vi "Laserpaneltcp.vi"() -> ()   [LabVIEW 2014]
uses:
  wlmData.dll
panel:
  out "Boolean 2":bool
  out "Boolean":bool
  in  "Warning 3":bool
  in  "Warning 2":bool
  in  "Warning 1":bool
  in  "Warning 0":bool
  out "Set Volt Array 0":dbl[](array[numeric])
  out "935":string
  out "729":string
  out "399":string
  out "370":string
  out "Act Wavelength number (nm)":dbl=70.0 format="%.6f"
  out "Set wave Array":dbl[](array[numeric])
  out "Lock Array":bool[](array[boolean])
  in  "stop":bool
  in  "Tab Control":enum32{"Laser Controller", "Wavelenth Meter"}(tab)
  out "Act Temperature":dbl=70.0 format="%.3f"
  out "Max Current (mA)":dbl=70.0 format="%.3f"
  out "Act Current (mA)":dbl=70.0 format="%.1f"
  in  "Set Wavelength (nm)":dbl=935.1882 format="%.6f"
  in  "Lock":bool
  in  "Laser":i16(ring) items=["370", "399", "729", "935"]
  out "Act Voltage (V)":dbl=70.0 format="%.3f"
  in  "Set Temperature":dbl=70.0 format="%.3f"
  in  "Set Current  (mA)":dbl=70.0 format="%.3f"
  in  "Set Voltage (V)":dbl=70.0 format="%.3f"
  out "Warning":bool
  in  "PID gains":T1={"proportional gain (Kc)"=1000.0, "integral time (Ti, min)"=0.0, "derivative time (Td, min)"=0.0} {"derivative time (Td, min)" format="%.3f"; "integral time (Ti, min)" format="%.3f"; "proportional gain (Kc)" format="%.3f"}
  out "Act Wavelength (nm)":string
  in  "PID Warning":bool
  in  "stop 3":bool
  in  "Use":bool=TRUE
  in  "Use":bool=TRUE
  in  "Use":bool=TRUE
  in  "Use":bool=TRUE
  in  "Expo.4[ms]":i32[](array[numeric])
  in  "Expo.3[ms]":i32[](array[numeric])
  in  "Expo.2[ms]":i32[](array[numeric])
  out "935 2":string
  out "729  2":string
  out "399 2":string
  out "370 2":string
  in  "Show":bool=TRUE
  in  "Show":bool=TRUE
  in  "Show":bool=TRUE
  in  "Show":bool=TRUE
  in  "Automatic":bool
  in  "Automatic":bool
  in  "Automatic":bool
  in  "Automatic":bool
  out "Pattern2":i16[][](graph)
  out "Pattern":i16[][](graph)
  in  "Expo.1[ms]":i32[](array[numeric])
  in  "stop 2":bool
  in  "Show WLM APP":bool=TRUE
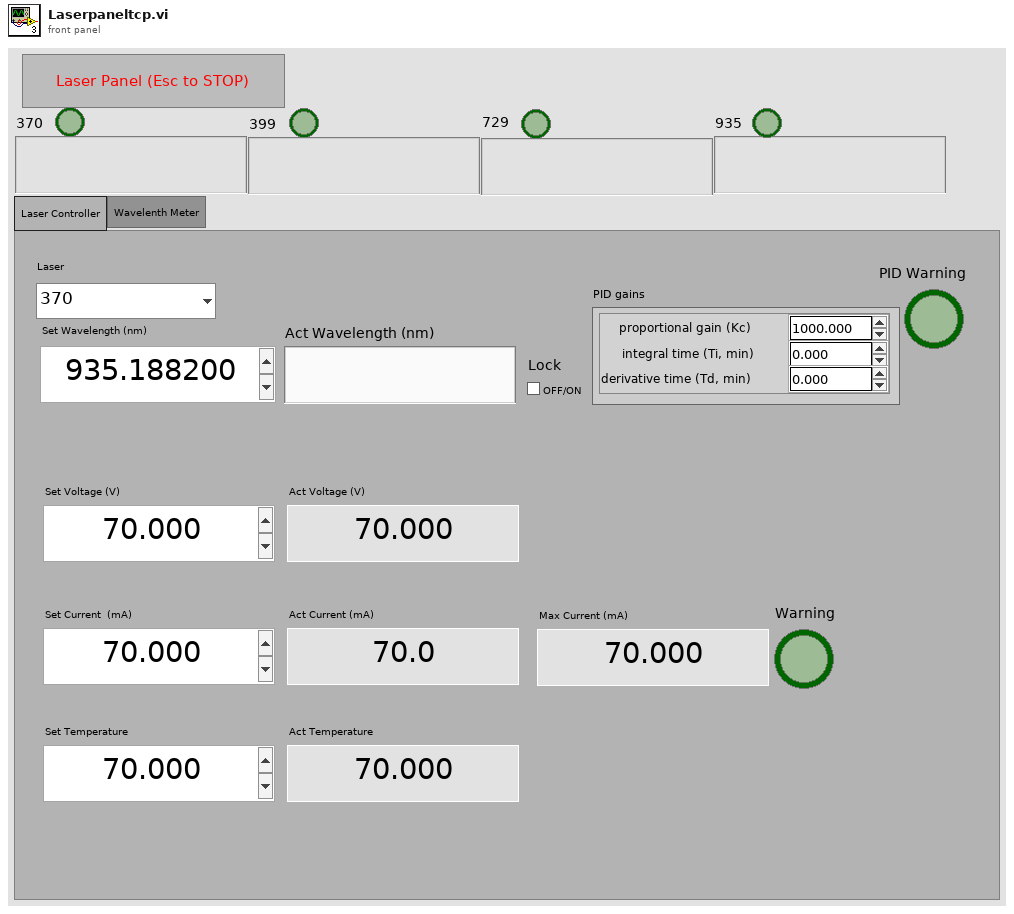
[diagram p1: front panel]
types:
  T1 = cluster{"proportional gain (Kc)":dbl, "integral time (Ti, min)":dbl, "derivative time (Td, min)":dbl}
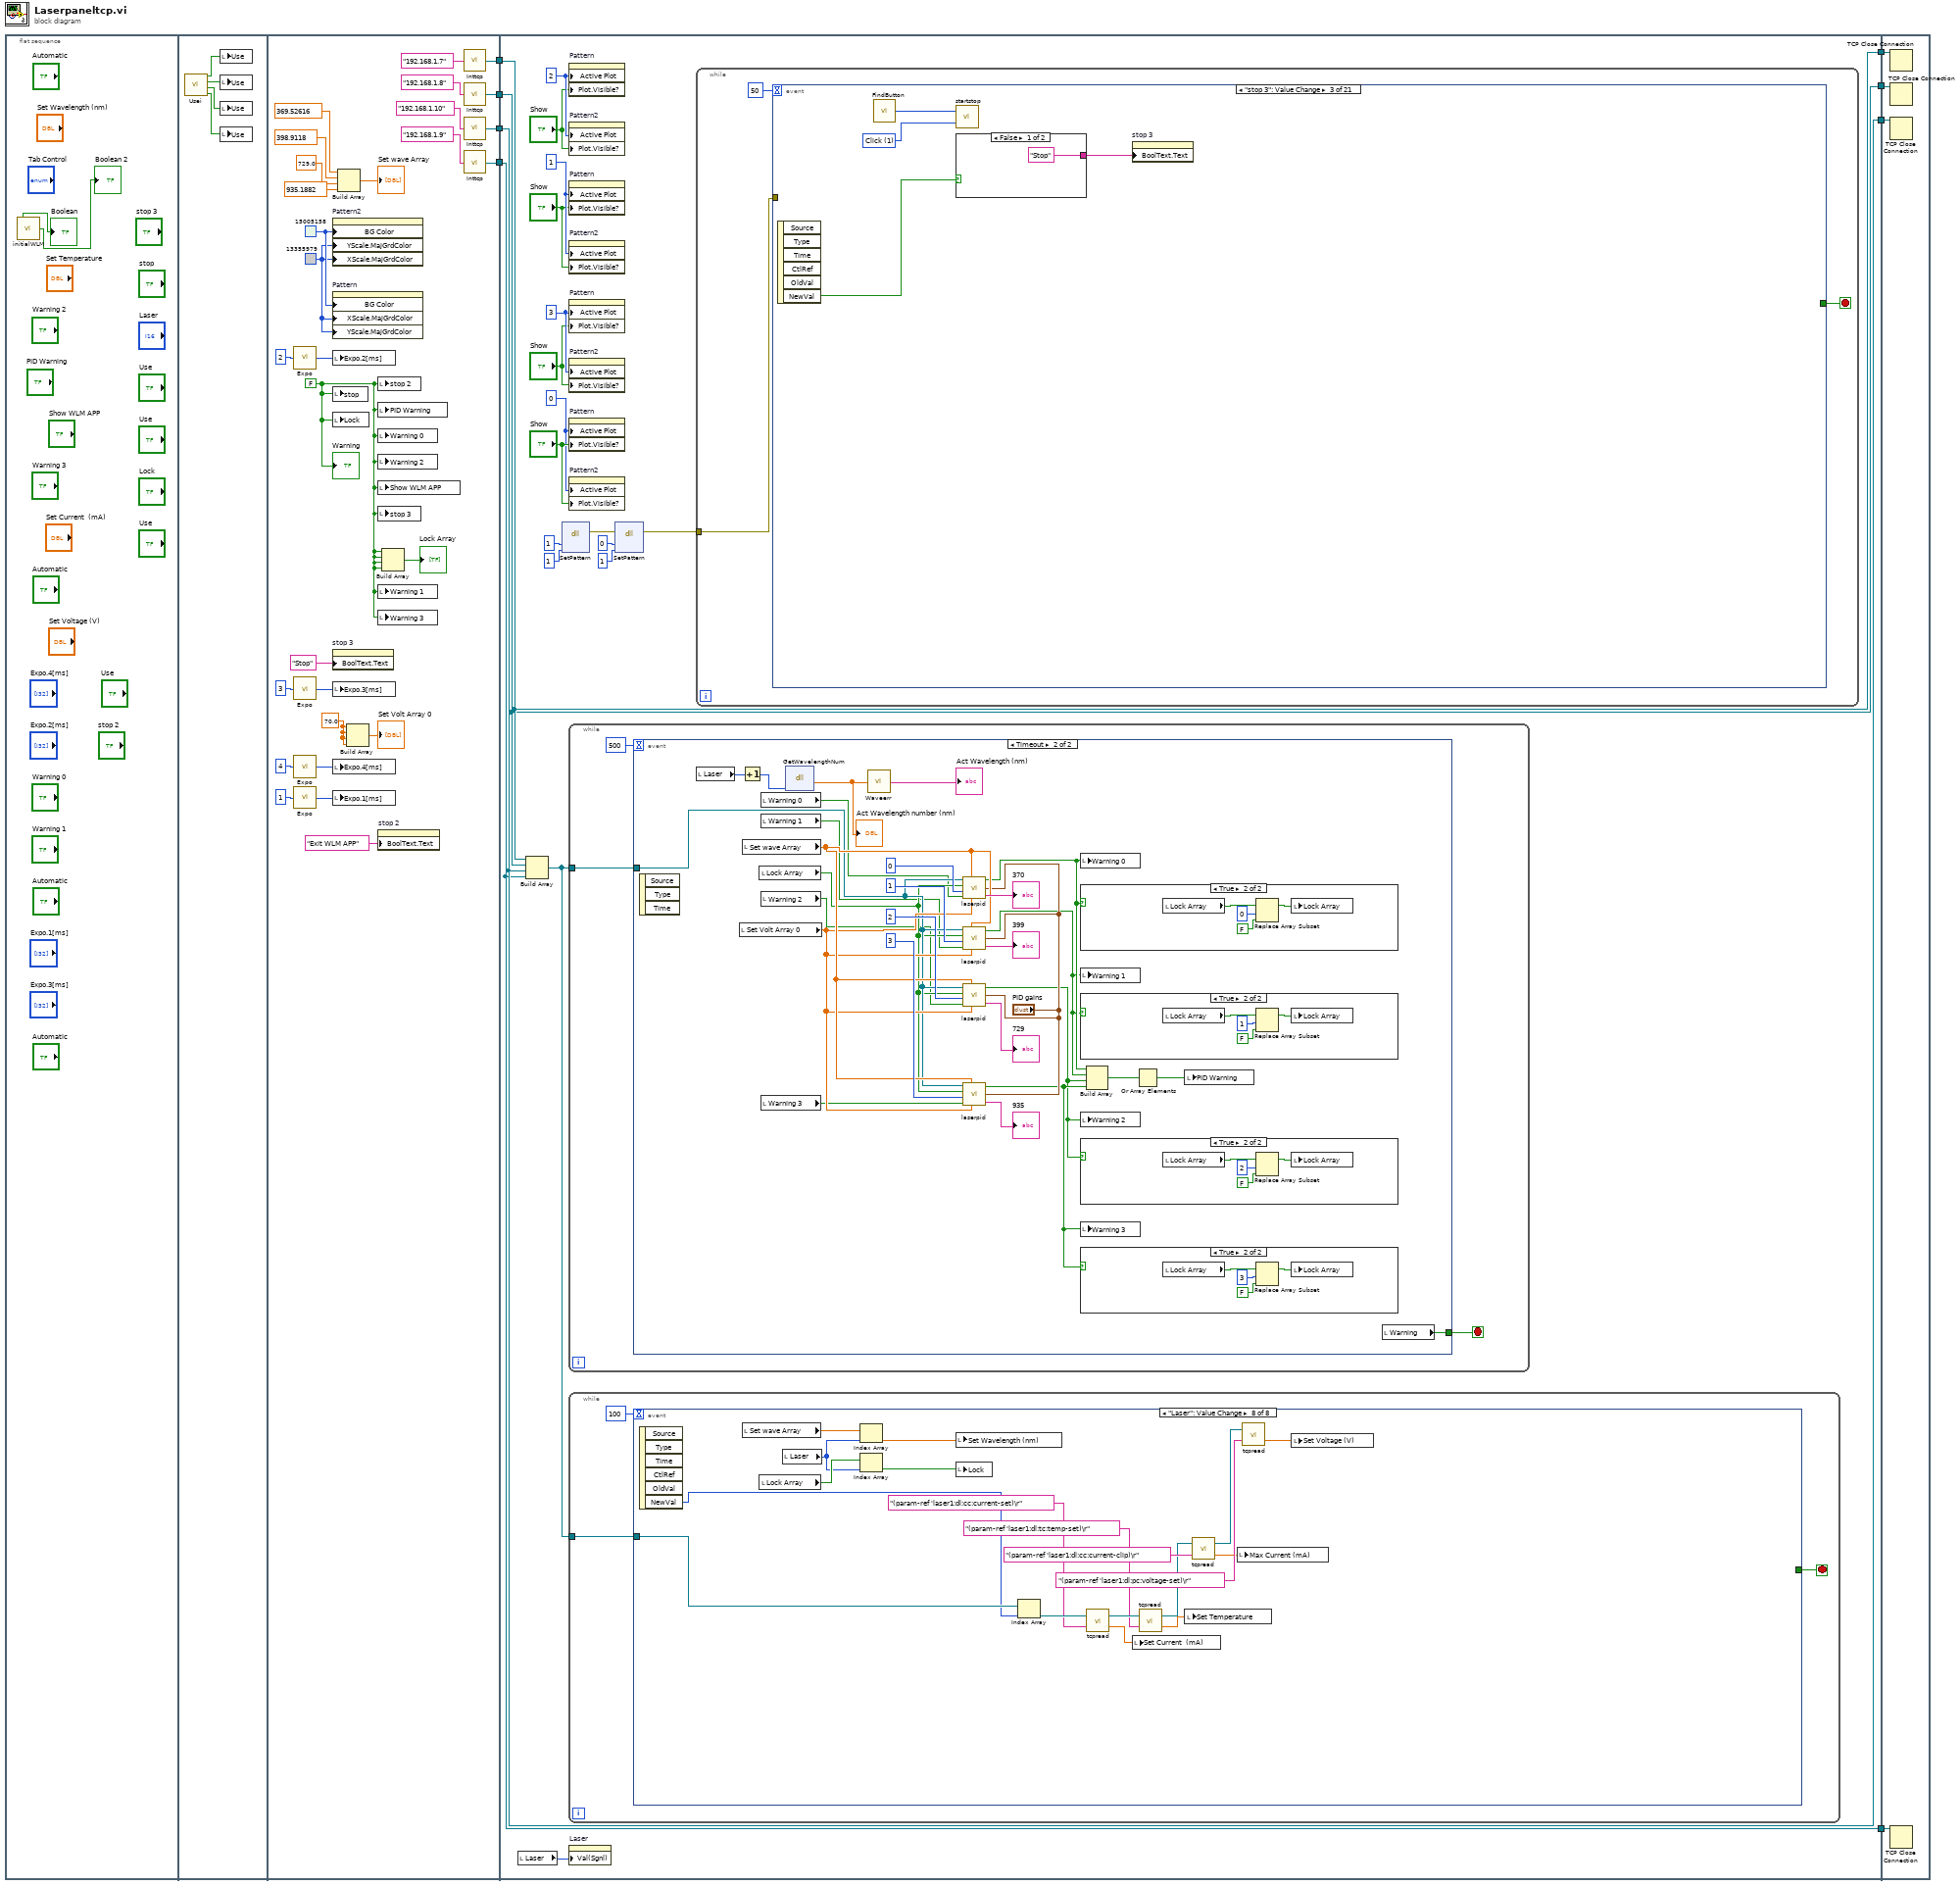
[diagram p0: block diagram]
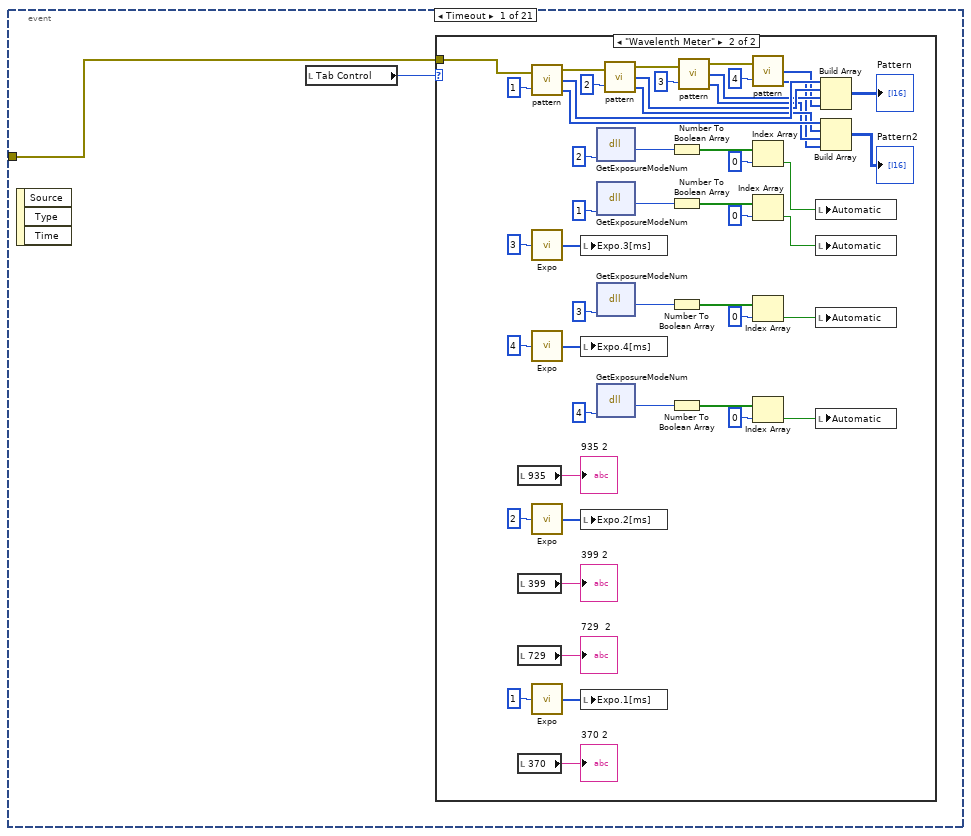
[diagram p2: hidden frame]
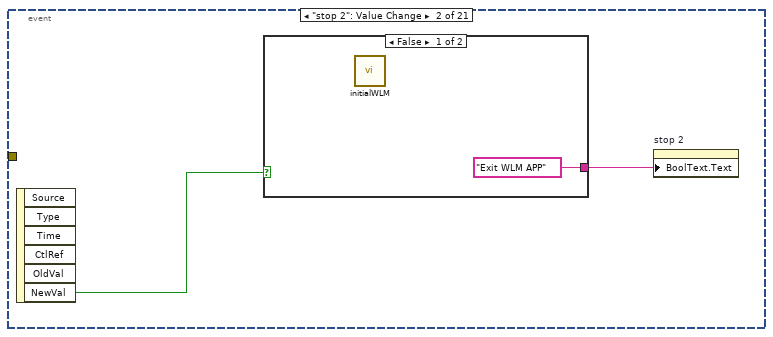
[diagram p4: hidden frame]
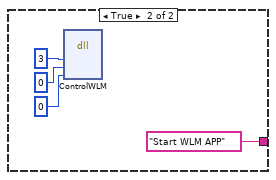
[diagram p5: hidden frame]
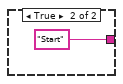
[diagram p6: hidden frame]
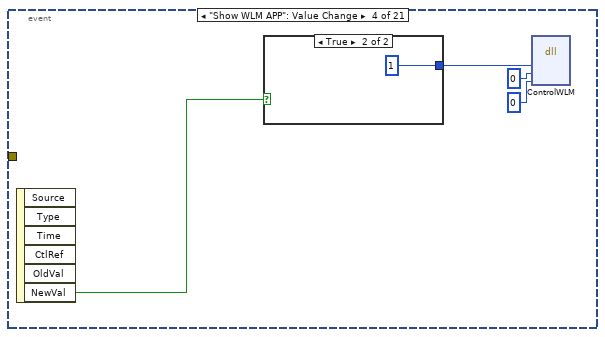
[diagram p7: hidden frame]
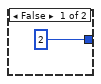
[diagram p8: hidden frame]
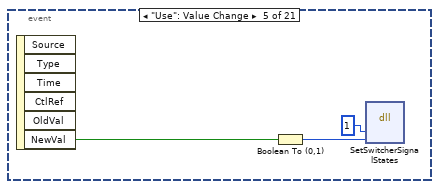
[diagram p9: hidden frame]
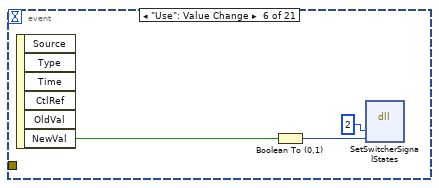
[diagram p10: hidden frame]
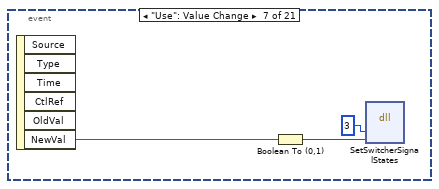
[diagram p11: hidden frame]
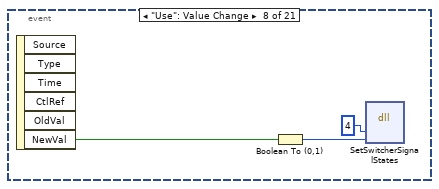
[diagram p12: hidden frame]
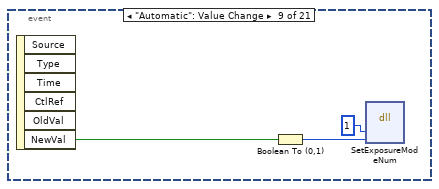
[diagram p13: hidden frame]
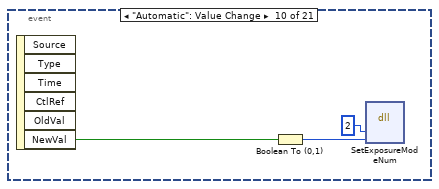
[diagram p14: hidden frame]
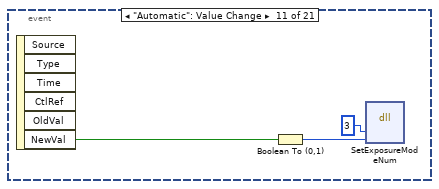
[diagram p15: hidden frame]
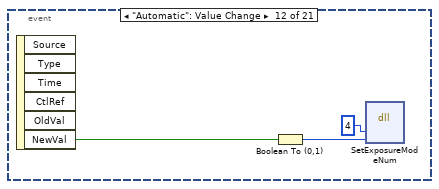
[diagram p16: hidden frame]
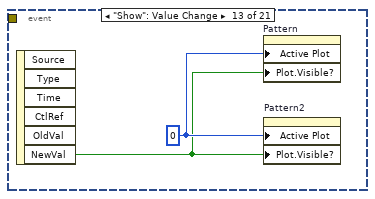
[diagram p17: hidden frame]
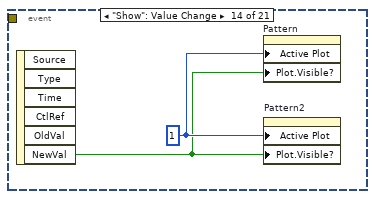
[diagram p18: hidden frame]
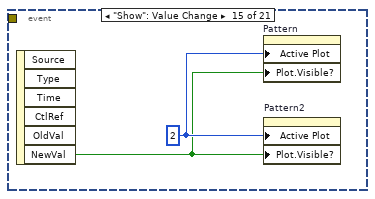
[diagram p19: hidden frame]
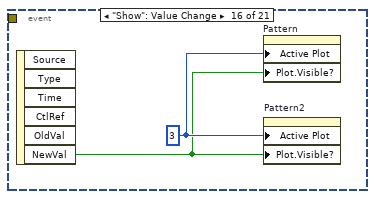
[diagram p20: hidden frame]
diagram:
  n1 = flat-sequence {
    tunnel: [w41] -> w8
    tunnel: [w40] -> w7
    tunnel: [w39] -> w6
    tunnel: [w38] -> w5
    tunnel: w8 -> [w62]
    tunnel: w7 -> [w61]
    tunnel: w6 -> [w60]
    tunnel: w5 -> [w59]
    tunnel: [w62] -> w4
    tunnel: [w61] -> w3
    tunnel: [w60] -> w2
    tunnel: [w59] -> w1
    tunnel: w4 -> [w360]
    tunnel: w3 -> [w359]
    tunnel: w2 -> [w358]
    tunnel: w1 -> [w357]
    frame #0 {
      n2 = call "initialWLM.vi"() -> ("Boolean 2"=→"Boolean 2":bool, "Boolean"=→"Boolean":bool)
    }
    frame #1 {
      n3 = call "Usei.vi"() -> ("Boolean 4"=w14:bool, "Boolean 3"=w13:bool, "Boolean 2"=w12:bool, "Boolean"=w11:bool)
      n4 = local write "Use"(w11) -> ()
      n5 = local write "Use"(w12) -> ()
      n6 = local write "Use"(w13) -> ()
      n7 = local write "Use"(w14) -> ()
    }
    frame #2 {
      w26 = u32 13355979 ("Color Box")
      w27 = u32 15005158
      w30 = 70.0
      w17 = FALSE
      n8 = call "Expo.vi"("Numeric"=2) -> ("Array"=w22:i32[])
      n9 = call "Expo.vi"("Numeric"=3) -> ("Array"=w20:i32[])
      n10 = call "Expo.vi"("Numeric"=4) -> ("Array"=w18:i32[])
      n11 = call "Expo.vi"("Numeric"=1) -> ("Array"=w24:i32[])
      n12 = property on="Pattern2" class="WFGraph (strict)"("BG Color"=w27, "YScale.MajGrdColor"=w26, "XScale.MajGrdColor"=w26) -> ()  [unwired: 2 in, 2 out]
      n13 = property on="Pattern" class="WFGraph (strict)"("BG Color"=w27, "XScale.MajGrdColor"=w26, "YScale.MajGrdColor"=w26) -> ()  [unwired: 2 in, 2 out]
      n14 = local write "Expo.2[ms]"(w22) -> ()
      n15 = local write "stop"(w17) -> ()
      n16 = local write "Lock"(w17) -> ()
      n17 = property on="stop 3" class="Bool (strict)"("BoolText.Text"="Stop") -> ()  [unwired: 2 in, 2 out]
      n18 = local write "Expo.3[ms]"(w20) -> ()
      n19 = local write "Expo.4[ms]"(w18) -> ()
      n20 = local write "Expo.1[ms]"(w24) -> ()
      n21 = Build Array(369.52616, 398.9118, 729.0, 935.1882) -> (→"Set wave Array":dbl[])
      n22 = Build Array(w30, w30, w30, w30) -> (→"Set Volt Array 0":dbl[])
      n23 = local write "stop 2"(w17) -> ()
      n24 = local write "PID Warning"(w17) -> ()
      n25 = local write "Warning 0"(w17) -> ()
      n26 = local write "Warning 2"(w17) -> ()
      n27 = local write "Show WLM APP"(w17) -> ()
      n28 = local write "stop 3"(w17) -> ()
      n29 = local write "Warning 1"(w17) -> ()
      n30 = local write "Warning 3"(w17) -> ()
      n31 = property on="stop 2" class="Bool (strict)"("BoolText.Text"="Exit WLM APP") -> ()  [unwired: 2 in, 2 out]
      n32 = Build Array(w17, w17, w17, w17) -> (→"Lock Array":bool[])
      n33 = call "Inttcp.vi"("String"="192.168.1.7" ("address")) -> ("TCP Network Connection Refnum"=w41:refnum<k5>)
      n34 = call "Inttcp.vi"("String"="192.168.1.8" ("address")) -> ("TCP Network Connection Refnum"=w40:refnum<k5>)
      n35 = call "Inttcp.vi"("String"="192.168.1.10" ("address")) -> ("TCP Network Connection Refnum"=w39:refnum<k5>)
      n36 = call "Inttcp.vi"("String"="192.168.1.9" ("address")) -> ("TCP Network Connection Refnum"=w38:refnum<k5>)
      "Warning" <- w17
    }
    frame #3 {
      w55 = 3
      w57 = 2
      w51 = 1
      w52 = 0
      n37 = local read "Laser"() -> (w63:i16)
      n38 = Build Array(w62, w61, w60, w59) -> (w58:refnum<k5>[])
      n39 = dll-call lib="wlmData.dll" fn="SetPattern"("Index"=1, "enable"=1) -> (error out=w45:errorcluster)  [unwired: 6 in, 1 out]
      n40 = property on="Pattern" class="WFGraph (strict)"("Active Plot"=w57, "Plot.Visible?"="Show") -> ()  [unwired: 2 in, 2 out]
      n41 = property on="Pattern2" class="WFGraph (strict)"("Active Plot"=w57, "Plot.Visible?"="Show") -> ()  [unwired: 2 in, 2 out]
      n42 = property on="Pattern" class="WFGraph (strict)"("Active Plot"=w51, "Plot.Visible?"="Show") -> ()  [unwired: 2 in, 2 out]
      n43 = property on="Pattern2" class="WFGraph (strict)"("Active Plot"=w51, "Plot.Visible?"="Show") -> ()  [unwired: 2 in, 2 out]
      n44 = property on="Pattern" class="WFGraph (strict)"("Active Plot"=w55, "Plot.Visible?"="Show") -> ()  [unwired: 2 in, 2 out]
      n45 = property on="Pattern2" class="WFGraph (strict)"("Active Plot"=w55, "Plot.Visible?"="Show") -> ()  [unwired: 2 in, 2 out]
      n46 = property on="Pattern" class="WFGraph (strict)"("Active Plot"=w52, "Plot.Visible?"="Show") -> ()  [unwired: 2 in, 2 out]
      n47 = property on="Pattern2" class="WFGraph (strict)"("Active Plot"=w52, "Plot.Visible?"="Show") -> ()  [unwired: 2 in, 2 out]
      n48 = while {
        tunnel: w58 -> [w205]
        stop <- w206 stop-if-true
        n49 = event shown="[1] Timeout" {
          selector: _ -> [_ _]
          dyn-events: _ -> [_ _]
          timeout: 500 -> [_ _]
          tunnel: [w208 w219] -> w206
          tunnel: w205 -> [_ w222]
          event "stop": Value Change {
            n50 = event-data() -> ("NewVal"=w208:bool)  [unwired: 1 in, 5 out]
          }
          event Timeout {
            n51 = event-data() -> ()  [unwired: 1 in, 3 out]
            n52 = local read "Laser"() -> (w233:i16)
            n53 = local read "Set Volt Array 0"() -> (w223:dbl[])
            n54 = Increment(x=w233) -> (x+1=w234:i16)
            n55 = local read "Set wave Array"() -> (w224:dbl[])
            n56 = local read "Lock Array"() -> (w221:bool[])
            n57 = local read "Warning 0"() -> (w218:bool)
            n58 = local read "Warning 1"() -> (w217:bool)
            n59 = local read "Warning 2"() -> (w216:bool)
            n60 = local read "Warning 3"() -> (w215:bool)
            n61 = dll-call lib="wlmData.dll" fn="GetWavelengthNum"("channel"=w234) -> ("res"=w235:dbl)  [unwired: 4 in, 2 out]
            "Act Wavelength number (nm)" <- w235
            n62 = call "Waveerr.vi"("Numeric"=w235) -> ("String"=→"Act Wavelength (nm)":string)
            n63 = call "laserpid.vi"("TCP Array"=w222, "Set wave Array"=w224, "Lock Array"=w221, "Numeric"=0, "Set volt Array 0"=w223, "waring in"=w218, "PID gains"="PID gains") -> ("warning out"=w214:bool, "wavelenth"=→"370":string)
            n64 = call "laserpid.vi"("TCP Array"=w222, "Set wave Array"=w224, "Lock Array"=w221, "Numeric"=1, "Set volt Array 0"=w223, "waring in"=w217, "PID gains"="PID gains") -> ("warning out"=w213:bool, "wavelenth"=→"399":string)
            n65 = call "laserpid.vi"("TCP Array"=w222, "Set wave Array"=w224, "Lock Array"=w221, "Numeric"=2, "Set volt Array 0"=w223, "waring in"=w216, "PID gains"="PID gains") -> ("warning out"=w211:bool, "wavelenth"=→"729":string)
            n66 = call "laserpid.vi"("TCP Array"=w222, "Set wave Array"=w224, "Lock Array"=w221, "Numeric"=3, "Set volt Array 0"=w223, "waring in"=w215, "PID gains"="PID gains") -> ("warning out"=w212:bool, "wavelenth"=→"935":string)
            n67 = local write "Warning 0"(w214) -> ()
            n68 = case shown="True" w214 {
              frame False {
              }
              frame True {
                n69 = local read "Lock Array"() -> (w243:bool[])
                n70 = Replace Array Subset(array=w243, new element=FALSE, index=0) -> (w242:bool[])
                n71 = local write "Lock Array"(w242) -> ()
              }
            }
            n72 = local write "Warning 1"(w213) -> ()
            n73 = case shown="True" w213 {
              frame False {
              }
              frame True {
                n74 = local read "Lock Array"() -> (w251:bool[])
                n75 = Replace Array Subset(array=w251, new element=FALSE, index=1) -> (w250:bool[])
                n76 = local write "Lock Array"(w250) -> ()
              }
            }
            n77 = local write "Warning 2"(w211) -> ()
            n78 = case shown="True" w211 {
              frame False {
              }
              frame True {
                n79 = local read "Lock Array"() -> (w248:bool[])
                n80 = Replace Array Subset(array=w248, new element=FALSE, index=2) -> (w247:bool[])
                n81 = local write "Lock Array"(w247) -> ()
              }
            }
            n82 = local write "Warning 3"(w212) -> ()
            n83 = case shown="True" w212 {
              frame False {
              }
              frame True {
                n84 = local read "Lock Array"() -> (w240:bool[])
                n85 = Replace Array Subset(array=w240, new element=FALSE, index=3) -> (w239:bool[])
                n86 = local write "Lock Array"(w239) -> ()
              }
            }
            n87 = Build Array(w214, w213, w211, w212) -> (w210:bool[])
            n88 = Or Array Elements(Boolean array=w210) -> (logical OR=w209:bool)
            n89 = local write "PID Warning"(w209) -> ()
            n90 = local read "Warning"() -> (w219:bool)
          }
        }
      }
      n91 = while {
        tunnel: w58 -> [w253]
        stop <- w255 stop-if-true
        n92 = event shown="[7] \"Laser\": Value Change" {
          selector: _ -> [_ _ _ _ _ _ _ _]
          dyn-events: _ -> [_ _ _ _ _ _ _ _]
          timeout: 100 -> [_ _ _ _ _ _ _ _]
          tunnel: [w256 _ w270 _ _ _ _ _] -> w255
          tunnel: w253 -> [_ w259 w279 w284 _ w322 w331 w356]
          event "stop": Value Change {
            n93 = event-data() -> ("NewVal"=w256:bool)  [unwired: 1 in, 5 out]
          }
          event "Set Voltage (V)": Value Change {
            n94 = event-data() -> ("NewVal"=w261:dbl)  [unwired: 1 in, 5 out]
            n95 = Number To Fractional String(number=w261) -> (F-format string=w264:string)  [unwired: 3 in]
            n96 = local read "Laser"() -> (w260:i16)
            n97 = Concatenate Strings("(param-set! 'laser1:dl:pc:voltage-set " ("string"), w264, ")" ("string"), "\n") -> (w257:string)
            n98 = Index Array(array=w259, index=w260) -> (element=w258:refnum<k5>)
            n99 = call "tcpread.vi"("String 2"=w257, "TCP Network Connection Refnum"=w258) -> ()  [unwired: 2 out]
          }
          event Timeout {
            n100 = event-data() -> ()  [unwired: 1 in, 3 out]
            n101 = local read "Laser"() -> (w280:i16)
            n102 = Index Array(array=w279, index=w280) -> (element=w269:refnum<k5>)
            n103 = call "tcpread.vi"("String 2"="(param-ref 'laser1:dl:cc:current-clip)\r", "TCP Network Connection Refnum"=w269) -> ("OUT"=w266:dbl, "TCP Network Connection Refnum 2"=w268:refnum<k5>)
            "Max Current (mA)" <- w266
            n104 = call "tcpread.vi"("String 2"="(param-ref 'laser1:dl:cc:current-act)\r" ("write buffer"), "TCP Network Connection Refnum"=w268) -> ("OUT"=w267:dbl, "TCP Network Connection Refnum 2"=w277:refnum<k5>)
            "Act Current (mA)" <- w267
            n105 = call "tcpread.vi"("String 2"="(param-ref 'laser1:dl:tc:temp-act)\r" ("write buffer"), "TCP Network Connection Refnum"=w277) -> ("OUT"=→"Act Temperature":dbl, "TCP Network Connection Refnum 2"=w274:refnum<k5>)
            n106 = Greater?(x=w267, y=w266) -> (0:w270:bool)
            n107 = local write "Warning"(w270) -> ()
            n108 = call "tcpread.vi"("String 2"="(param-ref 'laser1:dl:pc:voltage-act)\r" ("write buffer"), "TCP Network Connection Refnum"=w274) -> ("OUT"=→"Act Voltage (V)":dbl)  [unwired: 1 out]
          }
          event "Lock": Value Change {
            n109 = event-data() -> ("NewVal"=w286:bool)  [unwired: 1 in, 5 out]
            n110 = local read "Act Wavelength number (nm)"() -> (w288:dbl)
            n111 = local read "Laser"() -> (w283:i16)
            n112 = case shown="True" w286 {
              tunnel: w283 -> [_ w289]
              frame False {
              }
              frame True {
                n113 = flat-sequence {
                  tunnel: w289 -> [w291]
                  frame #0 {
                    n114 = case shown="0, Default" w291 {
                      tunnel: FALSE -> [w292 w293 w294 w295]
                      frame 0, Default {
                        n115 = local write "Warning 0"(w292) -> ()
                      }
                      frame 1 {
                        n116 = local write "Warning 1"(w293) -> ()
                      }
                      frame 2 {
                        n117 = local write "Warning 2"(w294) -> ()
                      }
                      frame 3 {
                        n118 = local write "Warning 3"(w295) -> ()
                      }
                    }
                  }
                  frame #1 {
                    n119 = local read "Warning 0"() -> (w299:bool)
                    n120 = local read "Warning 1"() -> (w297:bool)
                    n121 = local read "Warning 2"() -> (w298:bool)
                    n122 = local read "Warning 3"() -> (w296:bool)
                    n123 = Build Array(w299, w297, w298, w296) -> (w300:bool[])
                    n124 = Or Array Elements(Boolean array=w300) -> (logical OR=w301:bool)
                    n125 = local write "PID Warning"(w301) -> ()
                  }
                }
              }
            }
            n126 = Index Array(array=w284, index=w283) -> (element=w282:refnum<k5>)
            n127 = Greater Than 0?(x=w288) -> (x > 0?=w287:bool)
            n128 = case shown="True" w287 {
              tunnel: w286 -> [_ w306]
              tunnel: w283 -> [_ w303]
              frame False {
                n129 = local write "Lock"(FALSE) -> ()
              }
              frame True {
                n130 = flat-sequence {
                  tunnel: w303 -> [w307]
                  tunnel: w306 -> [w308]
                  tunnel: [w308] -> w305
                  tunnel: [w307] -> w304
                  tunnel: w305 -> [w313]
                  tunnel: w304 -> [w312]
                  frame #0 {
                    n131 = local read "Set Volt Array 0"() -> (w309:dbl[])
                    n132 = local read "Set Voltage (V)"() -> (w310:dbl)
                    n133 = Replace Array Subset(array=w309, new element=w310, index=w307) -> (w311:dbl[])
                    n134 = local write "Set Volt Array 0"(w311) -> ()
                  }
                  frame #1 {
                    n135 = local read "Lock Array"() -> (w315:bool[])
                    n136 = Replace Array Subset(array=w315, new element=w313, index=w312) -> (w314:bool[])
                    n137 = local write "Lock Array"(w314) -> ()
                  }
                }
              }
            }
            n138 = call "tcpread.vi"("String 2"="(param-ref 'laser1:dl:pc:voltage-set)\r" ("write buffer"), "TCP Network Connection Refnum"=w282) -> ("OUT"=w281:dbl)  [unwired: 1 out]
            n139 = local write "Set Voltage (V)"(w281) -> ()
          }
          event "Set Wavelength (nm)": Value Change {
            n140 = event-data() -> ("NewVal"=w319:dbl)  [unwired: 1 in, 5 out]
            n141 = local read "Set wave Array"() -> (w316:dbl[])
            n142 = local read "Laser"() -> (w317:i16)
            n143 = Replace Array Subset(array=w316, new element=w319, index=w317) -> (w318:dbl[])
            n144 = local write "Set wave Array"(w318) -> ()
          }
          event "Set Current  (mA)": Value Change {
            n145 = event-data() -> ("NewVal"=w324:dbl)  [unwired: 1 in, 5 out]
            n146 = Number To Fractional String(number=w324) -> (F-format string=w326:string)  [unwired: 3 in]
            n147 = local read "Laser"() -> (w323:i16)
            n148 = Concatenate Strings("(param-set! 'laser1:dl:cc:current-set " ("string"), w326, ")" ("string"), "\n") -> (w320:string)
            n149 = Index Array(array=w322, index=w323) -> (element=w321:refnum<k5>)
            n150 = call "tcpread.vi"("String 2"=w320, "TCP Network Connection Refnum"=w321) -> ()  [unwired: 2 out]
          }
          event "Set Temperature": Value Change {
            n151 = event-data() -> ("NewVal"=w333:dbl)  [unwired: 1 in, 5 out]
            n152 = Number To Fractional String(number=w333) -> (F-format string=w336:string)  [unwired: 3 in]
            n153 = local read "Laser"() -> (w332:i16)
            n154 = Concatenate Strings("(param-set! 'laser1:dl:tc:temp-set " ("string"), w336, ")" ("string"), "\n") -> (w329:string)
            n155 = Index Array(array=w331, index=w332) -> (element=w330:refnum<k5>)
            n156 = call "tcpread.vi"("String 2"=w329, "TCP Network Connection Refnum"=w330) -> ()  [unwired: 2 out]
          }
          event "Laser": Value Change {
            n157 = event-data() -> ("NewVal"=w355:i16)  [unwired: 1 in, 5 out]
            n158 = local read "Set wave Array"() -> (w339:dbl[])
            n159 = local read "Lock Array"() -> (w342:bool[])
            n160 = local read "Laser"() -> (w338:i16)
            n161 = Index Array(array=w339, index=w338) -> (element=w340:dbl)
            n162 = Index Array(array=w342, index=w338) -> (element=w341:bool)
            n163 = local write "Set Wavelength (nm)"(w340) -> ()
            n164 = local write "Lock"(w341) -> ()
            n165 = Index Array(array=w356, index=w355) -> (element=w354:refnum<k5>)
            n166 = call "tcpread.vi"("String 2"="(param-ref 'laser1:dl:cc:current-set)\r" ("write buffer"), "TCP Network Connection Refnum"=w354) -> ("OUT"=w352:dbl, "TCP Network Connection Refnum 2"=w351:refnum<k5>)
            n167 = local write "Set Current  (mA)"(w352) -> ()
            n168 = call "tcpread.vi"("String 2"="(param-ref 'laser1:dl:tc:temp-set)\r" ("write buffer"), "TCP Network Connection Refnum"=w351) -> ("OUT"=w349:dbl, "TCP Network Connection Refnum 2"=w344:refnum<k5>)
            n169 = local write "Set Temperature"(w349) -> ()
            n170 = call "tcpread.vi"("String 2"="(param-ref 'laser1:dl:cc:current-clip)\r", "TCP Network Connection Refnum"=w344) -> ("OUT"=w345:dbl, "TCP Network Connection Refnum 2"=w343:refnum<k5>)
            n171 = local write "Max Current (mA)"(w345) -> ()
            n172 = call "tcpread.vi"("String 2"="(param-ref 'laser1:dl:pc:voltage-set)\r" ("write buffer"), "TCP Network Connection Refnum"=w343) -> ("OUT"=w347:dbl)  [unwired: 1 out]
            n173 = local write "Set Voltage (V)"(w347) -> ()
          }
        }
      }
      n174 = property on="Laser" class="Ring (strict)"("Val(Sgnl)"=w63) -> ()  [unwired: 2 in, 2 out]
      n175 = dll-call lib="wlmData.dll" fn="SetPattern"(error in=w45, "Index"=0, "enable"=1) -> (error out=w44:errorcluster)  [unwired: 5 in, 1 out]
      n176 = while {
        tunnel: w44 -> [w64]
        stop <- w66 stop-if-true
        n177 = event shown="[2] \"stop 3\": Value Change" {
          selector: _ -> [_ _ _ _ _ _ _ _ _ _ _ _ _ _ _ _ _ _ _ _ _]
          dyn-events: _ -> [_ _ _ _ _ _ _ _ _ _ _ _ _ _ _ _ _ _ _ _ _]
          timeout: 50 -> [_ _ _ _ _ _ _ _ _ _ _ _ _ _ _ _ _ _ _ _ _]
          tunnel: [_ _ _ _ _ _ _ _ _ _ _ _ _ _ _ _ _ _ _ _ w178] -> w66
          tunnel: w64 -> [w67 _ _ _ _ _ _ _ _ _ _ _ _ _ _ _ _ _ _ _ _]
          event Timeout {
            n178 = event-data() -> ()  [unwired: 1 in, 3 out]
            n179 = local read "Tab Control"() -> (w68:enum32{"Laser Controller", "Wavelenth Meter"})
            n180 = case shown="\"Wavelenth Meter\"" w68 {
              tunnel: w67 -> [_ w69]
              frame "Laser Controller", Default {
              }
              frame "Wavelenth Meter" {
                n181 = local read "935"() -> (→"935 2":string)
                n182 = local read "399"() -> (→"399 2":string)
                n183 = local read "729"() -> (→"729  2":string)
                n184 = local read "370"() -> (→"370 2":string)
                n185 = call "pattern.vi"("Error In"=w69, "Numeric"=1) -> ("Error Out"=w72:errorcluster, "Pattern"=w110:i16[], "Pattern 2"=w109:i16[])
                n186 = call "Expo.vi"("Numeric"=3) -> ("Array"=w76:i32[])
                n187 = call "Expo.vi"("Numeric"=4) -> ("Array"=w78:i32[])
                n188 = call "Expo.vi"("Numeric"=2) -> ("Array"=w74:i32[])
                n189 = call "Expo.vi"("Numeric"=1) -> ("Array"=w79:i32[])
                n190 = local write "Expo.3[ms]"(w76) -> ()
                n191 = local write "Expo.4[ms]"(w78) -> ()
                n192 = local write "Expo.2[ms]"(w74) -> ()
                n193 = local write "Expo.1[ms]"(w79) -> ()
                n194 = dll-call lib="wlmData.dll" fn="GetExposureModeNum"("num"=2) -> ("res"=w97:i32)  [unwired: 4 in, 2 out]
                n195 = dll-call lib="wlmData.dll" fn="GetExposureModeNum"("num"=1) -> ("res"=w117:i32)  [unwired: 4 in, 2 out]
                n196 = dll-call lib="wlmData.dll" fn="GetExposureModeNum"("num"=3) -> ("res"=w94:i32)  [unwired: 4 in, 2 out]
                n197 = dll-call lib="wlmData.dll" fn="GetExposureModeNum"("num"=4) -> ("res"=w89:i32)  [unwired: 4 in, 2 out]
                n198 = call "pattern.vi"("Error In"=w72, "Numeric"=2) -> ("Error Out"=w71:errorcluster, "Pattern"=w107:i16[], "Pattern 2"=w106:i16[])
                n199 = Number To Boolean Array(number=w97) -> (Boolean array=w98:bool[])
                n200 = Number To Boolean Array(number=w117) -> (Boolean array=w116:bool[])
                n201 = Number To Boolean Array(number=w94) -> (Boolean array=w93:bool[])
                n202 = Number To Boolean Array(number=w89) -> (Boolean array=w90:bool[])
                n203 = call "pattern.vi"("Error In"=w71, "Numeric"=3) -> ("Error Out"=w70:errorcluster, "Pattern"=w103:i16[], "Pattern 2"=w101:i16[])
                n204 = call "pattern.vi"("Error In"=w70, "Numeric"=4) -> ("Pattern"=w102:i16[], "Pattern 2"=w100:i16[])  [unwired: 1 out]
                n205 = Index Array(array=w98, index=0) -> (element=w85:bool)
                n206 = Index Array(array=w116, index=0) -> (element=w115:bool)
                n207 = Index Array(array=w93, index=0) -> (element=w86:bool)
                n208 = Index Array(array=w90, index=0) -> (element=w87:bool)
                n209 = local write "Automatic"(w85) -> ()
                n210 = local write "Automatic"(w115) -> ()
                n211 = local write "Automatic"(w86) -> ()
                n212 = local write "Automatic"(w87) -> ()
                n213 = Build Array(w110, w107, w103, w102) -> (→"Pattern":i16[][])
                n214 = Build Array(w109, w106, w101, w100) -> (→"Pattern2":i16[][])
              }
            }
          }
          event "stop 2": Value Change {
            n215 = event-data() -> ("NewVal"=w120:bool)  [unwired: 1 in, 5 out]
            n216 = case shown="False" w120 {
              tunnel: ["Exit WLM APP" "Start WLM APP"] -> w119
              frame False {
                n217 = call "initialWLM.vi"() -> ()  [unwired: 2 out]
              }
              frame True {
                n218 = dll-call lib="wlmData.dll" fn="ControlWLM"("action"=3, "app"=0, "ver"=0) -> ()  [unwired: 7 in, 2 out]
              }
            }
            n219 = property on="stop 2" class="Bool (strict)"("BoolText.Text"=w119) -> ()  [unwired: 2 in, 2 out]
          }
          event "stop 3": Value Change {
            w128 = u16 1 items=["GetText", "Click"] ("Message")
            n220 = event-data() -> ("NewVal"=w127:bool)  [unwired: 1 in, 5 out]
            n221 = call "FindButton.vi"() -> ("Handle"=w129:u64)
            n222 = call "startstop.vi"("Message"=w128, "Handle"=w129) -> ()  [unwired: 1 in, 1 out]
            n223 = case shown="False" w127 {
              tunnel: ["Stop" "Start"] -> w126
              frame False {
              }
              frame True {
              }
            }
            n224 = property on="stop 3" class="Bool (strict)"("BoolText.Text"=w126) -> ()  [unwired: 2 in, 2 out]
          }
          event "Show WLM APP": Value Change {
            n225 = event-data() -> ("NewVal"=w133:bool)  [unwired: 1 in, 5 out]
            n226 = case shown="True" w133 {
              tunnel: [2 1] -> w132
              frame False {
              }
              frame True {
              }
            }
            n227 = dll-call lib="wlmData.dll" fn="ControlWLM"("action"=w132, "app"=0, "ver"=0) -> ()  [unwired: 7 in, 2 out]
          }
          event "Use": Value Change {
            n228 = event-data() -> ("NewVal"=w140:bool)  [unwired: 1 in, 5 out]
            n229 = Boolean To (0,1)(Boolean=w140) -> (0, 1=w138:i16)
            n230 = dll-call lib="wlmData.dll" fn="SetSwitcherSignalStates"("channel"=1, "use"=w138) -> ()  [unwired: 6 in, 2 out]
          }
          event "Use": Value Change {
            n231 = event-data() -> ("NewVal"=w141:bool)  [unwired: 1 in, 5 out]
            n232 = Boolean To (0,1)(Boolean=w141) -> (0, 1=w142:i16)
            n233 = dll-call lib="wlmData.dll" fn="SetSwitcherSignalStates"("channel"=2, "use"=w142) -> ()  [unwired: 6 in, 2 out]
          }
          event "Use": Value Change {
            n234 = event-data() -> ("NewVal"=w144:bool)  [unwired: 1 in, 5 out]
            n235 = Boolean To (0,1)(Boolean=w144) -> (0, 1=w145:i16)
            n236 = dll-call lib="wlmData.dll" fn="SetSwitcherSignalStates"("channel"=3, "use"=w145) -> ()  [unwired: 6 in, 2 out]
          }
          event "Use": Value Change {
            n237 = event-data() -> ("NewVal"=w147:bool)  [unwired: 1 in, 5 out]
            n238 = Boolean To (0,1)(Boolean=w147) -> (0, 1=w148:i16)
            n239 = dll-call lib="wlmData.dll" fn="SetSwitcherSignalStates"("channel"=4, "use"=w148) -> ()  [unwired: 6 in, 2 out]
          }
          event "Automatic": Value Change {
            n240 = event-data() -> ("NewVal"=w151:bool)  [unwired: 1 in, 5 out]
            n241 = Boolean To (0,1)(Boolean=w151) -> (0, 1=w150:i16)
            n242 = dll-call lib="wlmData.dll" fn="SetExposureModeNum"("num"=1, "Enable"=w150) -> ()  [unwired: 6 in, 2 out]
          }
          event "Automatic": Value Change {
            n243 = event-data() -> ("NewVal"=w153:bool)  [unwired: 1 in, 5 out]
            n244 = Boolean To (0,1)(Boolean=w153) -> (0, 1=w154:i16)
            n245 = dll-call lib="wlmData.dll" fn="SetExposureModeNum"("num"=2, "Enable"=w154) -> ()  [unwired: 6 in, 2 out]
          }
          event "Automatic": Value Change {
            n246 = event-data() -> ("NewVal"=w156:bool)  [unwired: 1 in, 5 out]
            n247 = Boolean To (0,1)(Boolean=w156) -> (0, 1=w157:i16)
            n248 = dll-call lib="wlmData.dll" fn="SetExposureModeNum"("num"=3, "Enable"=w157) -> ()  [unwired: 6 in, 2 out]
          }
          event "Automatic": Value Change {
            n249 = event-data() -> ("NewVal"=w159:bool)  [unwired: 1 in, 5 out]
            n250 = Boolean To (0,1)(Boolean=w159) -> (0, 1=w160:i16)
            n251 = dll-call lib="wlmData.dll" fn="SetExposureModeNum"("num"=4, "Enable"=w160) -> ()  [unwired: 6 in, 2 out]
          }
          event "Show": Value Change {
            w163 = 0
            n252 = event-data() -> ("NewVal"=w162:bool)  [unwired: 1 in, 5 out]
            n253 = property on="Pattern" class="WFGraph (strict)"("Active Plot"=w163, "Plot.Visible?"=w162) -> ()  [unwired: 2 in, 2 out]
            n254 = property on="Pattern2" class="WFGraph (strict)"("Active Plot"=w163, "Plot.Visible?"=w162) -> ()  [unwired: 2 in, 2 out]
          }
          event "Show": Value Change {
            w165 = 1
            n255 = event-data() -> ("NewVal"=w164:bool)  [unwired: 1 in, 5 out]
            n256 = property on="Pattern" class="WFGraph (strict)"("Active Plot"=w165, "Plot.Visible?"=w164) -> ()  [unwired: 2 in, 2 out]
            n257 = property on="Pattern2" class="WFGraph (strict)"("Active Plot"=w165, "Plot.Visible?"=w164) -> ()  [unwired: 2 in, 2 out]
          }
          event "Show": Value Change {
            w167 = 2
            n258 = event-data() -> ("NewVal"=w166:bool)  [unwired: 1 in, 5 out]
            n259 = property on="Pattern" class="WFGraph (strict)"("Active Plot"=w167, "Plot.Visible?"=w166) -> ()  [unwired: 2 in, 2 out]
            n260 = property on="Pattern2" class="WFGraph (strict)"("Active Plot"=w167, "Plot.Visible?"=w166) -> ()  [unwired: 2 in, 2 out]
          }
          event "Show": Value Change {
            w169 = 3
            n261 = event-data() -> ("NewVal"=w168:bool)  [unwired: 1 in, 5 out]
            n262 = property on="Pattern" class="WFGraph (strict)"("Active Plot"=w169, "Plot.Visible?"=w168) -> ()  [unwired: 2 in, 2 out]
            n263 = property on="Pattern2" class="WFGraph (strict)"("Active Plot"=w169, "Plot.Visible?"=w168) -> ()  [unwired: 2 in, 2 out]
          }
          event "Expo.1[ms]": Value Change {
            n264 = event-data() -> ("NewVal"=w170:i32[])  [unwired: 1 in, 5 out]
            n265 = call "Expow.vi"("Expo1[ms]"=w170, "Numeric"=1) -> ()
          }
          event "Expo.2[ms]": Value Change {
            n266 = event-data() -> ("NewVal"=w172:i32[])  [unwired: 1 in, 5 out]
            n267 = call "Expow.vi"("Expo1[ms]"=w172, "Numeric"=2) -> ()
          }
          event "Expo.3[ms]": Value Change {
            n268 = event-data() -> ("NewVal"=w174:i32[])  [unwired: 1 in, 5 out]
            n269 = call "Expow.vi"("Expo1[ms]"=w174, "Numeric"=3) -> ()
          }
          event "Expo.4[ms]": Value Change {
            n270 = event-data() -> ("NewVal"=w176:i32[])  [unwired: 1 in, 5 out]
            n271 = call "Expow.vi"("Expo1[ms]"=w176, "Numeric"=4) -> ()
          }
          event "stop": Value Change {
            n272 = event-data() -> ("NewVal"=w180:bool)  [unwired: 1 in, 5 out]
            n273 = flat-sequence {
              tunnel: w180 -> [w181]
              tunnel: [w181] -> w179
              tunnel: w179 -> [w204]
              tunnel: [w204] -> w178
              frame #0 {
                n274 = local read "Boolean"() -> (w182:bool)
                n275 = case shown="False" w182 {
                  frame False {
                    n276 = dll-call lib="wlmData.dll" fn="ControlWLM"("action"=1, "app"=0, "ver"=0) -> ()  [unwired: 7 in, 2 out]
                    n277 = local read "Boolean 2"() -> (w186:bool)
                    n278 = case shown="False" w186 {
                      frame False {
                        w189 = u16 0 items=["GetText", "Click"] ("Message")
                        n279 = call "FindButton.vi"() -> ("Handle"=w187:u64)
                        n280 = call "startstop.vi"("Message"=w189, "Handle"=w187) -> ("Output"=w191:variant)  [unwired: 1 in]
                        n281 = Variant To Data(type="", Variant=w191) -> (data=w188:string)  [unwired: 1 in, 1 out]
                        n282 = case shown="\"&Stop\"" w188 {
                          tunnel: w187 -> [w192 _]
                          frame Default {
                            w193 = u16 1 items=["GetText", "Click"] ("Message")
                            n283 = call "startstop.vi"("Message"=w193, "Handle"=w192) -> ()  [unwired: 1 in, 1 out]
                          }
                          frame "&Stop" {
                          }
                        }
                      }
                      frame True {
                        w196 = u16 0 items=["GetText", "Click"] ("Message")
                        n284 = call "FindButton.vi"() -> ("Handle"=w194:u64)
                        n285 = call "startstop.vi"("Message"=w196, "Handle"=w194) -> ("Output"=w198:variant)  [unwired: 1 in]
                        n286 = Variant To Data(type="", Variant=w198) -> (data=w195:string)  [unwired: 1 in, 1 out]
                        n287 = case shown="\"&Start\"" w195 {
                          tunnel: w194 -> [w199 _]
                          frame Default {
                            w200 = u16 1 items=["GetText", "Click"] ("Message")
                            n288 = call "startstop.vi"("Message"=w200, "Handle"=w199) -> ()  [unwired: 1 in, 1 out]
                          }
                          frame "&Start" {
                          }
                        }
                      }
                    }
                  }
                  frame True {
                    n289 = dll-call lib="wlmData.dll" fn="ControlWLM"("action"=3, "app"=0, "ver"=0) -> ()  [unwired: 7 in, 2 out]
                  }
                }
              }
              frame #1 {
              }
            }
          }
        }
      }
    }
    frame #4 {
      n290 = TCP Close Connection(connection ID=w360) -> ()  [unwired: 2 in, 2 out]
      n291 = TCP Close Connection(connection ID=w359) -> ()  [unwired: 2 in, 2 out]
      n292 = TCP Close Connection(connection ID=w358) -> ()  [unwired: 2 in, 2 out]
      n293 = TCP Close Connection(connection ID=w357) -> ()  [unwired: 2 in, 2 out]
    }
  }
